vi "setOffset.vi"(8 "error in (no error)":errorcluster, 10 "Offset Mode":T1=enum."Remove", 11 "Instrument.Lockin in":refnum<class "Instrument.Lockin.lvclass">) -> (0 "error out":errorcluster, 3 "Instrument.Lockin out":refnum<class "Instrument.Lockin.lvclass">)   [LabVIEW 2019, in "Instrument.Lockin.lvclass"]
doc: "API to put lockin into IV mode.\n\nIf address=\"\", this API reads from localhost\nIf address is remote lockin, you need to add this computer to allowed whitelist on the lockin computer you are trying to access."
uses:
  Instrument.Lockin.lvclass
  Typedefs/Offset Mode--Enum.ctl
  C:/Program Files (x86)/National Instruments/LabVIEW 2019/user.lib/LevyLab/Instrument Framework/SMOs/Instrument/Instrument.lvclass
  Typedefs/API/Lockin.Commands--Enum.ctl
  <userlib>/LevyLab/Instrument Framework/SMOs/Instrument/Instrument.lvclass/Instrument.ctl
  dce59797-926e-44ff-adbc-0402ea62d6fc.vi
  dce59797-926e-44ff-adbc-0402ea62d6fc.vi/046cd2dd-3af2-4e98-93c3-0971ea31d5e0.vi
  dce59797-926e-44ff-adbc-0402ea62d6fc.vi/046cd2dd-3af2-4e98-93c3-0971ea31d5e0.vi/2db0098d-e14c-4009-a7f6-0f6a8aea8d13.vi
  <userlib>/LevyLab/Instrument Framework/SMOs/Instrument/API/Send and Receive.vi
  dce59797-926e-44ff-adbc-0402ea62d6fc.vi/046cd2dd-3af2-4e98-93c3-0971ea31d5e0.vi/e14a9888-d92a-4162-8321-822a01ce508d.vi
  <userlib>/LevyLab/Instrument Framework/SMOs/Instrument/Private/Get Client Type.vi
  dce59797-926e-44ff-adbc-0402ea62d6fc.vi/046cd2dd-3af2-4e98-93c3-0971ea31d5e0.vi/2db0098d-e14c-4009-a7f6-0f6a8aea8d13.vi/e83fb8ab-ece5-47fd-901f-3abd5a5ee809.vi
  dce59797-926e-44ff-adbc-0402ea62d6fc.vi/046cd2dd-3af2-4e98-93c3-0971ea31d5e0.vi/2db0098d-e14c-4009-a7f6-0f6a8aea8d13.vi/74925fac-dd8f-4c0e-a394-2e68876da230.vi
  dce59797-926e-44ff-adbc-0402ea62d6fc.vi/046cd2dd-3af2-4e98-93c3-0971ea31d5e0.vi/e14a9888-d92a-4162-8321-822a01ce508d.vi/36dbc0b0-1775-4b3e-b1f8-da2689f4fd5b.vi
  dce59797-926e-44ff-adbc-0402ea62d6fc.vi/046cd2dd-3af2-4e98-93c3-0971ea31d5e0.vi/e14a9888-d92a-4162-8321-822a01ce508d.vi/d48a2905-58ef-4c5b-898f-aac75f44d48f.vi
  dce59797-926e-44ff-adbc-0402ea62d6fc.vi/046cd2dd-3af2-4e98-93c3-0971ea31d5e0.vi/e14a9888-d92a-4162-8321-822a01ce508d.vi/36dbc0b0-1775-4b3e-b1f8-da2689f4fd5b.vi/465c96c0-6cdf-434f-84cc-73fe17e4ecb5.vi
  dce59797-926e-44ff-adbc-0402ea62d6fc.vi/046cd2dd-3af2-4e98-93c3-0971ea31d5e0.vi/e14a9888-d92a-4162-8321-822a01ce508d.vi/36dbc0b0-1775-4b3e-b1f8-da2689f4fd5b.vi/220ca67f-c243-484f-9509-0a864c00ea2d.vi
  <userlib>/LevyLab/Instrument Framework/SMOs/Instrument/Private/Get RC Connection Status.vi
  <userlib>/LevyLab/Instrument Framework/SMOs/Instrument/API/Enum to String.vi
  <userlib>/LevyLab/Instrument Framework/SMOs/RemoteControl/API/Send and Receive.vi
  <vilib>/Utility/Data Type/Get Type Information.vi
  <vilib>/JDP Science/JSONtext/JSON text to Variant.vi
  <userlib>/LevyLab/Instrument Framework/SMOs/Instrument/API/Instrument.GetPublicEvents.vi
  <vilib>/JDP Science/JSONtext/Variant to JSON Text.vi
  <vilib>/National Instruments/GUID Generator/Guid Generator.vi
  <userlib>/LevyLab/Instrument Framework/SMOs/Instrument/API/Instrument.MessageToProcess.vi
  <userlib>/LevyLab/Instrument Framework/SMOs/Instrument/Private/Instrument.MessageFromProcess.EventStructure.vi
  <vilib>/JDP Science/JSONtext/LVClass Serializer/JSONtext LVClass Serializer.lvclass
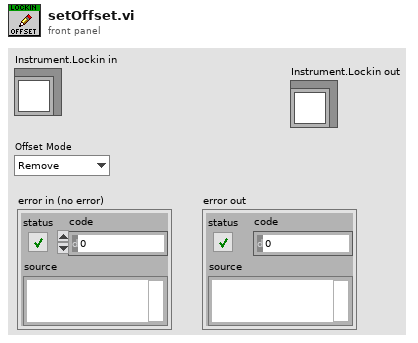
[diagram p1: front panel]
types:
  T1 = typedef "Instrument.Lockin.lvclass/Offset Mode--Enum.ctl" = enum16{"Measure", "Remove"}
  T2 = typedef "Instrument.Lockin.lvclass/Lockin.Commands--Enum.ctl" = enum16{"setAI", "setAO", "setAO_Amplitude", "setAO_DC", "setAO_Frequency", "setAO_Phase", "setAO_Function", "setAO_I+", "setREF", "setREF_Frequency", "setREF_Phase", "setREF_TC", "setREF_Roll-Off", "setDAQ", "setSampling", "setOffset", "setState", "getState", "getAO", "getAI", "getResults", "getSampling", "getAOconfig", "getREFconfig", "setInputGain", "setOutputGain", "getInputGain", "getOutputGain", "setSamplingMode", "getSamplingMode", "setSweep", "setSweepTime", "setSweepTable", "getStatus", "getSweepResults", "getSweepWaveforms", "startSweep", "stopSweep", "setAUX", "getAUX"}
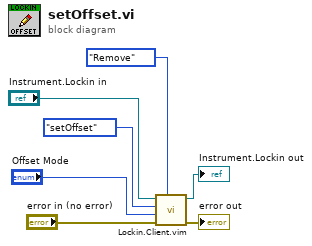
[diagram p0: block diagram]
diagram:
  n1 = call "Lockin.Client.vim"("Data Out type"=Offset_Mode--Enum."Remove" ("Offset Mode"), "error in (no error)"="error in (no error)", "Data"="Offset Mode", "Command"=Lockin.Commands--Enum."setOffset", "Instrument.Lockin in"="Instrument.Lockin in") -> ("error out"=→"error out":errorcluster, "Instrument.Lockin out"=→"Instrument.Lockin out":refnum<class "Instrument.Lockin.lvclass">)  [unwired: 4 in, 1 out]
